vi "4.vi"() -> ()   [LabVIEW 2021]
uses:
  1d7c82fd-b8af-4503-810e-330c205de7cb.vi
panel:
  out "deleted portion":i32
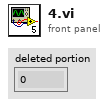
[diagram p1: front panel]
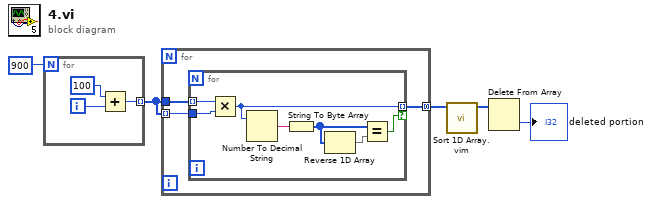
[diagram p0: block diagram]
diagram:
  n1 = for {
    N: 900 -> [_]
    tunnel: [w6] -> w4 mode=indexing
    i -> [w7]
    n2 = Add(x=100, y=w7) -> (x+y=w6:i32)
  }
  n3 = for {
    tunnel: w4 -> [w11]
    tunnel: w4 -> [w10] mode=indexing
    tunnel: [w9] -> w3 mode=concatenating
    n4 = for {
      tunnel: w11 -> [w18] mode=indexing
      tunnel: w10 -> [w17]
      tunnel: [w13] -> w9 mode=indexing if=w12
      n5 = Multiply(x=w18, y=w17) -> (x*y=w13:i32)
      n6 = Number To Decimal String(number=w13) -> (decimal integer string=w15:string)  [unwired: 1 in]
      n7 = String To Byte Array(string=w15) -> (unsigned byte array=w16:u8[])
      n8 = Reverse 1D Array(array=w16) -> (reversed array=w14:u8[])
      n9 = Equal?(x=w16, y=w14) -> (x = y?=w12:bool)
    }
  }
  n10 = call "Sort 1D Array.vim"("unsorted array"=w3) -> ("sorted array"=w2:i32[])  [unwired: 10 in]
  n11 = Delete From Array(array=w2) -> (deleted portion=→"deleted portion":i32)  [unwired: 2 in, 1 out]
